vi "shortcut_keys.vi"(5 "Cluster":T1) -> ()   [LabVIEW 2023]
panel:
  # "※スイッチ動作は4.Latch when pressedに設定"
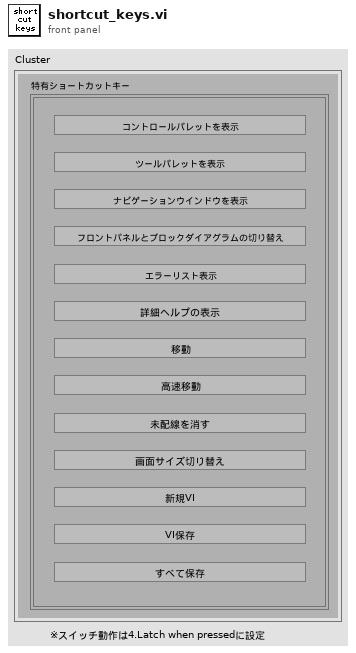
[diagram p1: front panel]
types:
  T1 = cluster{"ショートカットキー":bool, "ショートカットキー 2":bool, "ショートカットキー 3":bool, "ショートカットキー 4":bool, "ショートカットキー 5":bool, "ショートカットキー 6":bool, "ショートカットキー 7":bool, "ショートカットキー 8":bool, "ショートカットキー 9":bool, "ショートカットキー 10":bool, "ショートカットキー 11":bool, "ショートカットキー 12":bool, "ショートカットキー 13":bool}
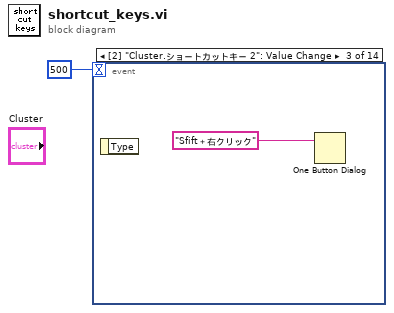
[diagram p0: block diagram]
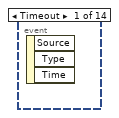
[diagram p2: hidden frame]
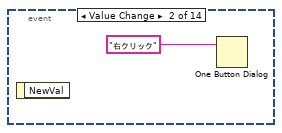
[diagram p3: hidden frame]
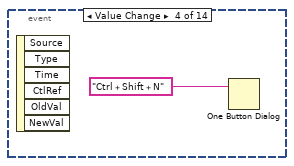
[diagram p4: hidden frame]
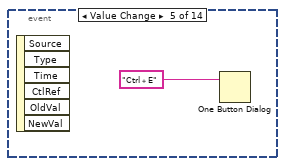
[diagram p5: hidden frame]
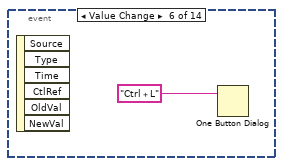
[diagram p6: hidden frame]
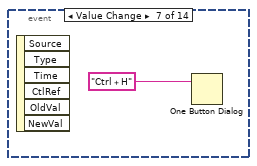
[diagram p7: hidden frame]
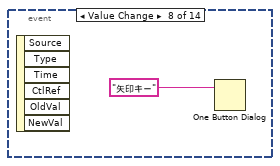
[diagram p8: hidden frame]
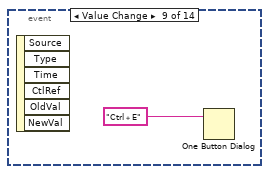
[diagram p9: hidden frame]
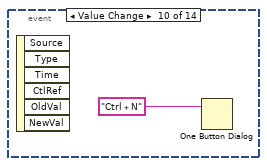
[diagram p10: hidden frame]
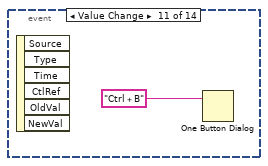
[diagram p11: hidden frame]
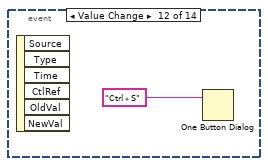
[diagram p12: hidden frame]
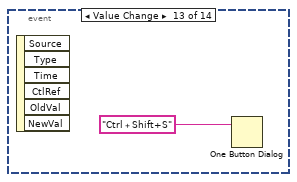
[diagram p13: hidden frame]
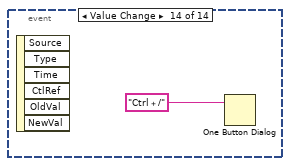
[diagram p14: hidden frame]
diagram:
  n1 = event shown="[2] \"Cluster.ショートカットキー 2\": Value Change" {
    selector: _ -> [_ _ _ _ _ _ _ _ _ _ _ _ _ _]
    dyn-events: _ -> [_ _ _ _ _ _ _ _ _ _ _ _ _ _]
    timeout: 500 -> [_ _ _ _ _ _ _ _ _ _ _ _ _ _]
    event Timeout {
      n2 = event-data() -> ()  [unwired: 1 in, 3 out]
    }
    event "Cluster.ショートカットキー": Value Change {
      n3 = event-data() -> ()  [unwired: 1 in, 1 out]
      n4 = One Button Dialog(message="右クリック") -> ()  [unwired: 1 in, 1 out]
    }
    event "Cluster.ショートカットキー 2": Value Change {
      n5 = event-data() -> ()  [unwired: 1 in, 1 out]
      n6 = One Button Dialog(message="Sfift＋右クリック") -> ()  [unwired: 1 in, 1 out]
    }
    event "Cluster.ショートカットキー 3": Value Change {
      n7 = event-data() -> ()  [unwired: 1 in, 6 out]
      n8 = One Button Dialog(message="Ctrl＋Shift＋N") -> ()  [unwired: 1 in, 1 out]
    }
    event "Cluster.ショートカットキー 4": Value Change {
      n9 = event-data() -> ()  [unwired: 1 in, 6 out]
      n10 = One Button Dialog(message="Ctrl＋E") -> ()  [unwired: 1 in, 1 out]
    }
    event "Cluster.ショートカットキー 5": Value Change {
      n11 = event-data() -> ()  [unwired: 1 in, 6 out]
      n12 = One Button Dialog(message="Ctrl＋L") -> ()  [unwired: 1 in, 1 out]
    }
    event "Cluster.ショートカットキー 6": Value Change {
      n13 = event-data() -> ()  [unwired: 1 in, 6 out]
      n14 = One Button Dialog(message="Ctrl＋H") -> ()  [unwired: 1 in, 1 out]
    }
    event "Cluster.ショートカットキー 7": Value Change {
      n15 = event-data() -> ()  [unwired: 1 in, 6 out]
      n16 = One Button Dialog(message="矢印キー") -> ()  [unwired: 1 in, 1 out]
    }
    event "Cluster.ショートカットキー 8": Value Change {
      n17 = event-data() -> ()  [unwired: 1 in, 6 out]
      n18 = One Button Dialog(message="Ctrl＋E") -> ()  [unwired: 1 in, 1 out]
    }
    event "Cluster.ショートカットキー 9": Value Change {
      n19 = event-data() -> ()  [unwired: 1 in, 6 out]
      n20 = One Button Dialog(message="Ctrl＋N") -> ()  [unwired: 1 in, 1 out]
    }
    event "Cluster.ショートカットキー 10": Value Change {
      n21 = event-data() -> ()  [unwired: 1 in, 6 out]
      n22 = One Button Dialog(message="Ctrl＋B") -> ()  [unwired: 1 in, 1 out]
    }
    event "Cluster.ショートカットキー 11": Value Change {
      n23 = event-data() -> ()  [unwired: 1 in, 6 out]
      n24 = One Button Dialog(message="Ctrl＋S") -> ()  [unwired: 1 in, 1 out]
    }
    event "Cluster.ショートカットキー 12": Value Change {
      n25 = event-data() -> ()  [unwired: 1 in, 6 out]
      n26 = One Button Dialog(message="Ctrl＋Shift+S") -> ()  [unwired: 1 in, 1 out]
    }
    event "Cluster.ショートカットキー 13": Value Change {
      n27 = event-data() -> ()  [unwired: 1 in, 6 out]
      n28 = One Button Dialog(message="Ctrl＋/") -> ()  [unwired: 1 in, 1 out]
    }
  }
